vi "dR_R_for_ThemalImaging(SGL).vi"(10 "DR/R parameter":T2, 11 "数据值引用":refnum<data-value>) -> (3 "Image Dst Out":T1)   [LabVIEW 2011]
uses:
  <vilib>/vision/Image Controls.llb/IMAQ Image.ctl
  <vilib>/vision/NI_Vision_Development_Module.lvlib
panel:
  out "数组 2":bool[](array[boolean])
  out "Image":T1(plugin-control)
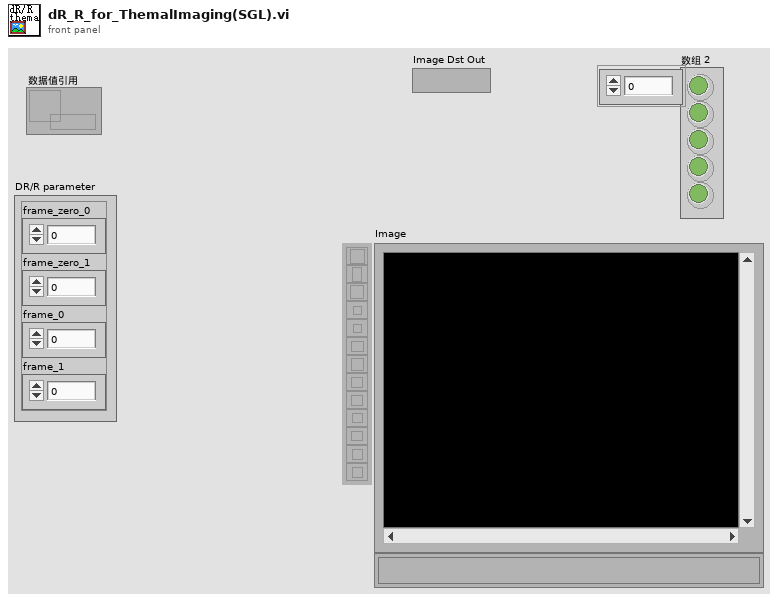
[diagram p1: front panel]
types:
  T1 = typedef "IMAQ Image.ctl" = refnum<image>
  T2 = cluster{"frame_zero_0":i32, "frame_zero_1":i32, "frame_0":i32, "frame_1":i32}
  T3 = typedef "Image Type" = u32
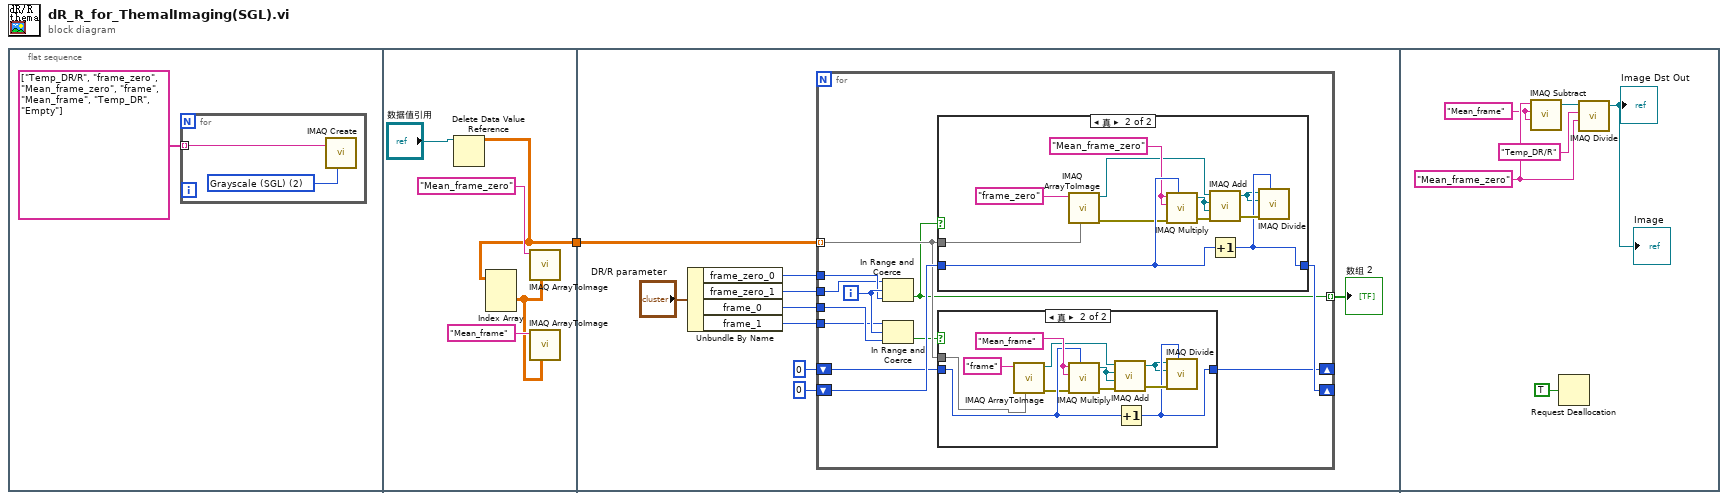
[diagram p0: block diagram]
diagram:
  n1 = flat-sequence {
    tunnel: [w5] -> w1
    tunnel: w1 -> [w10]
    frame #0 {
      n2 = for {
        tunnel: string[] ["Temp_DR/R", "frame_zero", "Mean_frame_zero", "frame", "Mean_frame", "Temp_DR", "Empty"] ("添加的数组") -> [w3] mode=indexing
        w4 = T3 2 items=["Grayscale (U8)", "Grayscale (I16)", "Grayscale (SGL)", "Complex (CSG)", "RGB (U32)", "HSL (U32)", "RGB (U64)", "Grayscale (U16)"] ("Image Type")
        n3 = call "IMAQ Create"("Image Name"=w3, "Image Type"=w4) -> ()  [unwired: 3 in, 2 out]
      }
    }
    frame #1 {
      n4 = Delete Data Value Reference(data value reference="数据值引用") -> (data value=w5:sgl[][][])  [unwired: 1 in, 1 out]
      n5 = Index Array(array=w5) -> (element=w7:sgl[][])  [unwired: 3 in]
      n6 = call "IMAQ ArrayToImage"("Image Pixels (Float)"=w7, "Image"="Mean_frame_zero" ("Image Name")) -> ()  [unwired: 8 in, 2 out]
      n7 = call "IMAQ ArrayToImage"("Image Pixels (Float)"=w7, "Image"="Mean_frame" ("Image Name")) -> ()  [unwired: 8 in, 2 out]
    }
    frame #2 {
      n8 = Unbundle By Name("DR/R parameter") -> ("frame_zero_0"=w17:i32, "frame_zero_1"=w16:i32, "frame_0"=w14:i32, "frame_1"=w13:i32)
      n9 = for {
        tunnel: w10 -> [w27] mode=indexing
        tunnel: w17 -> [w22]
        tunnel: w16 -> [w21]
        shift-right: [w29] -> _
        shift-left: 0 -> [w30]
        tunnel: w14 -> [w20]
        tunnel: w13 -> [w19]
        shift-right: [w25] -> _
        shift-left: 0 -> [w26]
        tunnel: [w23] -> w11 mode=indexing
        i -> [w28]
        n10 = In Range and Coerce(upper limit=w21, x=w28, lower limit=w22) -> (In Range?=w23:bool)  [unwired: 1 out]
        n11 = In Range and Coerce(upper limit=w19, x=w28, lower limit=w20) -> (In Range?=w24:bool)  [unwired: 1 out]
        n12 = case shown="真" w23 {
          tunnel: w27 -> [_ w54]
          tunnel: w30 -> [w43 w53]
          tunnel: [w43 w49] -> w29
          frame False {
          }
          frame True {
            w47 = "Mean_frame_zero" ("Image Name")
            n13 = call "IMAQ ArrayToImage"("Image Pixels (Float)"=w54, "Image"="frame_zero" ("Image Name")) -> ("error out"=w50:errorcluster, "Image Out"=w44:T1)  [unwired: 8 in]
            n14 = call "IMAQ Multiply"("Image Src A"=w47, "Constant"=w53, "Image Dst"=w47, "error in (no error)"=w50) -> ("Image Dst Out"=w45:T1, "error out"=w51:errorcluster)  [unwired: 3 in]
            n15 = call "IMAQ Add"("Image Src A"=w44, "Image Dst"=w45, "Image Src B"=w45, "error in (no error)"=w51) -> ("Image Dst Out"=w46:T1, "error out"=w52:errorcluster)  [unwired: 3 in]
            n16 = Increment(x=w53) -> (x+1=w49:i32)
            n17 = call "IMAQ Divide"("Image Src A"=w46, "Constant"=w49, "Image Dst"=w46, "error in (no error)"=w52) -> ()  [unwired: 3 in, 2 out]
          }
        }
        n18 = case shown="真" w24 {
          tunnel: w27 -> [_ w42]
          tunnel: w26 -> [w31 w39]
          tunnel: [w31 w33] -> w25
          frame False {
          }
          frame True {
            w40 = "Mean_frame" ("Image Name")
            n19 = call "IMAQ ArrayToImage"("Image Pixels (Float)"=w42, "Image"="frame" ("Image Name")) -> ("error out"=w34:errorcluster, "Image Out"=w38:T1)  [unwired: 8 in]
            n20 = call "IMAQ Multiply"("Image Src A"=w40, "Constant"=w39, "Image Dst"=w40, "error in (no error)"=w34) -> ("Image Dst Out"=w37:T1, "error out"=w35:errorcluster)  [unwired: 3 in]
            n21 = call "IMAQ Add"("Image Src A"=w38, "Image Dst"=w37, "Image Src B"=w37, "error in (no error)"=w35) -> ("Image Dst Out"=w32:T1, "error out"=w36:errorcluster)  [unwired: 3 in]
            n22 = Increment(x=w39) -> (x+1=w33:i32)
            n23 = call "IMAQ Divide"("Image Src A"=w32, "Constant"=w33, "Image Dst"=w32, "error in (no error)"=w36) -> ()  [unwired: 3 in, 2 out]
          }
        }
      }
      "数组 2" <- w11
    }
    frame #3 {
      w58 = "Mean_frame_zero" ("Image Name")
      w57 = "Mean_frame" ("Image Name")
      n24 = call "IMAQ Subtract"("Image Src A"=w58, "Image Dst"=w57, "Image Src B"=w57) -> ("Image Dst Out"=w60:T1)  [unwired: 4 in, 1 out]
      n25 = Request Deallocation(TRUE ("标志")) -> ()
      n26 = call "IMAQ Divide"("Image Src A"=w60, "Image Dst"="Temp_DR/R" ("Image Name"), "Image Src B"=w58) -> ("Image Dst Out"=→"Image Dst Out" →"Image":T1)  [unwired: 4 in, 1 out]
    }
  }
